vi "xcopyQAMTFiles.vi"(7 "error in (no error)":errorcluster, 8 "Destination":string="c:\\temp\n", 9 "SourceFile":string="IP10013LF_15-A150600262-RT3-1*.html", 10 "Machine":string="QAMT01") -> (0 "error out":errorcluster, 2 "concatenated string":string)   [LabVIEW 2012]
uses:
  <vilib>/addons/database/Connection.llb/DB Tools Open Connec (Path).vi
  <vilib>/addons/database/Connection.llb/Conn Execute.vi
  <vilib>/addons/database/Recordset.llb/Rec Fetch String Data (R).vi
  <vilib>/addons/database/Recordset.llb/Rec Destroy - Connection.vi
  <vilib>/addons/database/NI_Database_API.lvlib
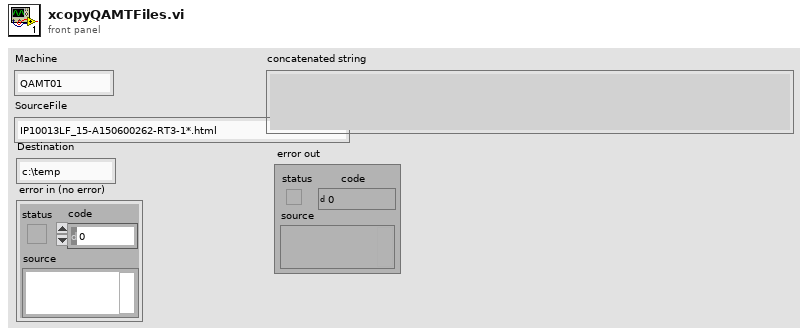
[diagram p1: front panel]
types:
  T1 = typedef "NI_Database_API.lvlib/Conn ObjectReference.ctl" = refnum<k1>
  T2 = typedef "NI_Database_API.lvlib/Rec ObjectReference.ctl" = refnum<k1>
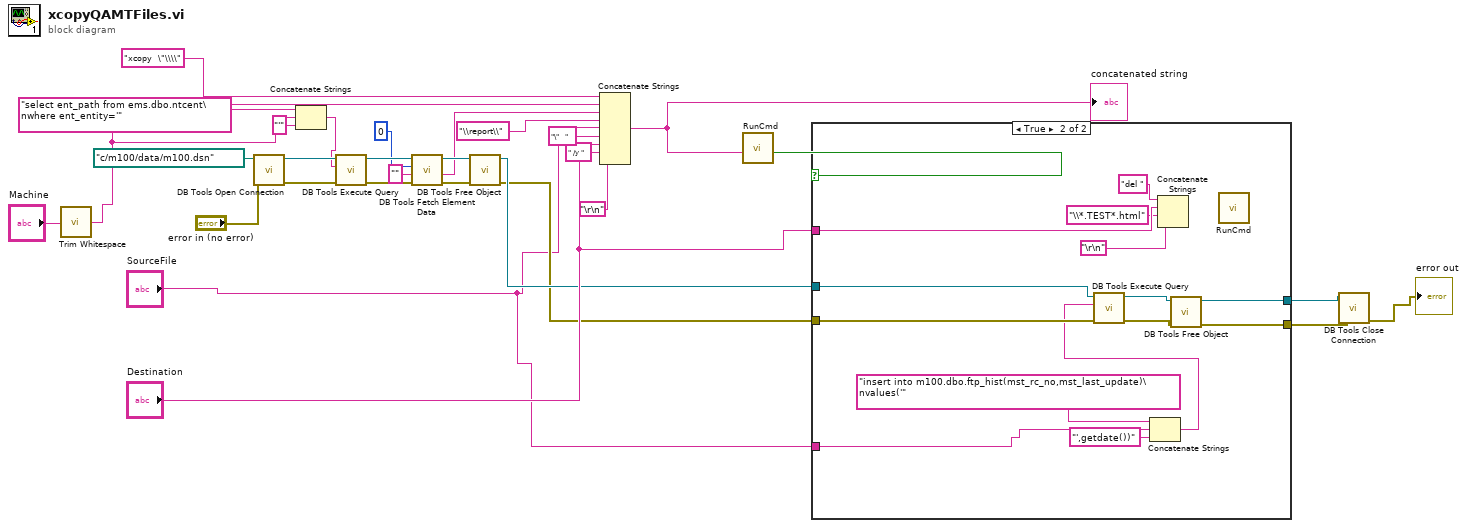
[diagram p0: block diagram]
diagram:
  n1 = call <vilib>:"Trim Whitespace.vi"("string"="Machine") -> ("trimmed string"=w21:string)  [unwired: 1 in]
  n2 = call-poly <vilib>:"DB Tools Open Connection.vi"("error in (no error)"="error in (no error)", "connection information"=path "c:/m100/data/m100.dsn") -> ("error out"=w29:errorcluster, "connection reference"=w30:T1)  [unwired: 6 in]
  n3 = Concatenate Strings("select ent_path from ems.dbo.ntcent\nwhere ent_entity='" ("string"), w21, "'" ("string")) -> (w19:string)
  n4 = call-poly <vilib>:"DB Tools Execute Query.vi"("error in (no error)"=w29, "SQL query"=w19, "connection reference"=w30) -> ("error out"=w27:errorcluster, "recordset reference"=w28:T2)  [unwired: 5 in]
  n5 = call-poly <vilib>:"DB Tools Fetch Element Data.vi"("error in (no error)"=w27, "type"="", "column index"=0, "recordset reference"=w28) -> ("error out"=w25:errorcluster, "data"=w16:string, "recordset reference out"=w26:T2)  [unwired: 3 in]
  n6 = call-poly <vilib>:"DB Tools Free Object.vi"("error in (no error)"=w25, "recordset reference"=w26) -> ("error out"=w7:errorcluster, "connection reference"=w8:T1)  [unwired: 8 in]
  n7 = Concatenate Strings("xcopy  \"\\\\" ("string"), w21, w16, "\\report\\" ("string"), "SourceFile", "\"   " ("string"), "Destination", " /y " ("string"), "\r\n") -> (w11:string)
  "concatenated string" <- w11
  n8 = call "RunCmd.vi"("Cmd String"=w11) -> ("OK"=w10:bool)  [unwired: 9 in, 1 out]
  n9 = case shown="True" w10 {
    tunnel: "Destination" -> [_ w45]
    tunnel: w8 -> [w32 w42]
    tunnel: w7 -> [w31 w41]
    tunnel: "SourceFile" -> [_ w39]
    tunnel: [w32 w34] -> w5
    tunnel: [w31 w33] -> w4
    frame False {
    }
    frame True {
      n10 = Concatenate Strings("insert into m100.dbo.ftp_hist(mst_rc_no,mst_last_update)\nvalues('" ("string"), w39, "',getdate())" ("string")) -> (w37:string)
      n11 = call-poly <vilib>:"DB Tools Execute Query.vi"("error in (no error)"=w41, "SQL query"=w37, "connection reference"=w42) -> ("error out"=w35:errorcluster, "recordset reference"=w36:T2)  [unwired: 5 in]
      n12 = Concatenate Strings("del " ("string"), w45, "\\*.TEST*.html" ("string"), "\r\n") -> ()  [unwired: 1 out]
      n13 = call-poly <vilib>:"DB Tools Free Object.vi"("error in (no error)"=w35, "recordset reference"=w36) -> ("error out"=w33:errorcluster, "connection reference"=w34:T1)  [unwired: 8 in]
      n14 = call "RunCmd.vi"() -> ()  [unwired: 10 in, 2 out]
    }
  }
  n15 = call <vilib>:"DB Tools Close Connection.vi"("error in (no error)"=w4, "connection reference"=w5) -> ("error out"=→"error out":errorcluster)  [unwired: 5 in]
